vi "Q14070-Z120主界面.vi"() -> ()   [LabVIEW 2013]
uses:
  PCI8622_32.dll
  <vilib>/printing/EasyPrintingControls.llb/report_type.ctl
  <vilib>/Utility/NIReport.llb/NI_ReportGenerationCore.lvlib
  <vilib>/printing/EasyPrintingControls.llb/contents.ctl
  <vilib>/Utility/NIReport.llb/NI_report.lvclass
  <vilib>/printing/EasyPrinting.llb/Easy Print VI Panel or Documentation (path).vi
panel:
  out "电压值":dbl format="%#_4g"
  out "右压力换向(N)":dbl=5000.0 format="%#.2f"
  out "左压力换向(N)":dbl=5000.0 format="%#.2f"
  out "右压力换向":bool
  out "左压力换向":bool
  out "气缸启用":dbl
  in  "型号数量":i32=2
  in  "光幕报警工步":dbl
  out "光幕报警提示":string
  out "顶升压力":dbl
  out "右伺服顶升位置":dbl format="%#.2f"
  out "左伺服顶升位置":dbl format="%#.2f"
  out "右顶升压力合格":bool
  out "左顶升压力合格":bool
  out "保压时间":dbl
  out "error out":errorcluster
  out "右伺服压入深度上限(mm)":dbl format="%#.2f"
  out "右伺服压入深度下限(mm)":dbl format="%#.2f"
  out "右伺服压入力上限(N)":dbl format="%#.2f"
  out "右伺服压入力下限(N)":dbl format="%#.2f"
  out "左伺服压入深度上限(mm)":dbl format="%#.2f"
  out "左伺服压入深度下限(mm)":dbl format="%#.2f"
  out "左伺服压入力上限(N)":dbl format="%#.2f"
  out "左伺服压入力下限(N)":dbl format="%#.2f"
  out "查询上序完成":bool
  out "上序合格":bool
  out "上序完成":bool
  out "本序完成":bool
  out "本序合格":bool
  in  "产品ID字符位数":dbl
  out "压力报警1":bool
  out "压力报警2":bool
  out "伺服慢进速度":dbl
  out "右伺服慢进位置":dbl format="%#.2f"
  out "左伺服慢进位置":dbl format="%#.2f"
  out "JSSJ":string
  out "FGCS":string
  out "KSSJ":string
  out "右压力参数组":dbl[](array[numeric])
  out "右位移参数组":dbl[](array[numeric])
  out "左压力参数组":dbl[](array[numeric])
  out "左位移参数组":dbl[](array[numeric])
  out "右伺服设定走位":dbl
  out "左伺服设定走位":dbl
  out "程序选择-2":bool
  out "程序选择-1":bool
  out "工步提示2":string
  out "工步提示1":string
  in  "报警工步号":u32 caption="工步号1"
  out "报警提示":string
  in  "自动工步号":u32 caption="工步号1"
  out "自动工步提示":string
  in  "产品ID":string="201209190001"
  out "员工ID":string
  out "员工姓名":string
  in  "电动缸全回零":bool
  in  "电动缸全复位":bool
  out "右伺服快进位置":dbl format="%#.2f"
  out "左伺服快进位置":dbl format="%#.2f"
  out "伺服快进速度":dbl
  out "参数保存错误":errorcluster
  out "传感器保存错误":errorcluster
  out "左实时压力(N)":dbl format="%#.3f"
  out "左实时位移(mm)":dbl=10000.0 format="%#.2f"
  out "右实时位移(mm)":dbl=10000.0 format="%#.2f"
  out "右实时压力(N)":dbl format="%#.3f"
  out "区域最小压力(N)":dbl format="%#.3f"
  out "监控点最大压力(N)":dbl format="%#.3f"
  out "监控点最小压力(N)":dbl format="%#.3f"
  out "区域最大压力(N)":dbl format="%#.3f"
  out "区域最小位移(mm)":dbl format="%#.1f"
  out "区域最大位移(mm)":dbl format="%#.1f"
  in  "左工步号2900":u32 caption="工步号1"
  in  "右工步号2700":u32 caption="工步号"
  in  "报警清除":bool
  in  "参数加载":bool
  in  "型号选择":u32(ring) items=["J706", "J709", "J728", "J728A", "J728B", "J506X"]
  out "参数加载错误":errorcluster
  in  "停止":bool
  out "ADODB._Connection Out":refnum<k7>
  out "参数查询错误":errorcluster
  in  "联线按钮":bool
  out "通讯状态":bool
  in  "选项卡控件":T1(tab)
  out "右区域最大压力(N)":dbl
  out "右区域最小压力(N)":dbl
  out "左区域最大压力(N)":dbl
  out "左区域最小压力(N)":dbl
  out "右实测压入压力(N)":dbl format="%#.1f"
  out "左实测压入压力(N)":dbl format="%#.1f"
  out "左压力位移曲线":cluster{"Y":dbl[], "Y":dbl[]}[](graph)=[{"Y"=array[221 elements], "Y"=array[221 elements]}, {"Y"=[130.0, 150.0, 150.0, 130.0, 130.0], "Y"=[0.0, 0.0, 4000.0, 4000.0, 0.0]}] caption="XY图"
  out "右压力位移曲线":cluster{"Y":dbl[], "Y":dbl[]}[](graph)=[{"Y"=array[234 elements], "Y"=array[234 elements]}, {"Y"=[130.0, 150.0, 150.0, 130.0, 130.0], "Y"=[0.0, 0.0, 4000.0, 4000.0, 0.0]}] caption="XY图"
  out "左实测监控点压力(N)":dbl format="%#.3f"
  out "左实测压入位移(mm)":dbl format="%#.1f"
  out "右实测压入位移(mm)":dbl format="%#.1f"
  out "右实测监控点压力(N)":dbl format="%#.3f"
  out "监控点位移(mm)":dbl format="%#.2f"
  out "左压装合格":bool
  out "左压装不合格":bool
  out "右压装不合格":bool
  out "右压装合格":bool
  out "右电动缸零位":bool
  out "左电动缸下限":bool
  out "右气缸下降":bool
  out "右气缸上升":bool
  out "右气缸下位":bool
  out "右气缸上位":bool
  out "左气缸上升":bool
  out "左气缸下降":bool
  out "左气缸上位":bool
  out "左气缸下位":bool
  out "左电动缸零位":bool
  out "右电动缸上限":bool
  out "右电动缸下限":bool
  out "左电动缸上限":bool
  in  "顶升气缸上升-右":bool
  in  "顶升气缸下降-右":bool
  in  "顶升气缸上升-左":bool
  in  "顶升气缸下降-左":bool
  out "启动2按钮":bool
  out "启动1按钮":bool
  out "手动/自动":bool
  out "复位按钮":bool
  in  "电动缸下降-右":bool
  in  "电动缸上升-右":bool
  in  "电动缸下降-左":bool
  in  "电动缸上升-左":bool
  in  "电动缸回零-右":bool
  in  "电动缸回零-左":bool
  in  "电动缸复位-左":bool
  in  "电动缸复位-右":bool
  out "急停按钮":bool
  out "安全光幕":bool
  out "气压报警":bool
  in  "光幕报警使能":bool
  in  "右伺服设定走位":dbl caption="右伺服设定走位负值"
  in  "左伺服设定走位":dbl caption="左伺服设定走位负值"
  in  "电动缸绝对移动调试-右":bool
  in  "电动缸绝对移动调试-左":bool
  out "左伺服实时位置":dbl
  out "右伺服实时位置":dbl
  in  "电动缸复位-右 2":bool
  in  "电动缸复位-左 2":bool
  in  "电动缸回零-左 2":bool
  in  "电动缸回零-右 2":bool
  in  "电动缸下降-右 2":bool
  in  "电动缸上升-右 2":bool
  in  "电动缸下降-左 2":bool
  in  "电动缸上升-左 2":bool
  out "J709减震套批次号输入成功":bool
  out "J706右减震套批次号输入成功":bool
  out "J706左减震套批次号输入成功":bool
  in  "J709减震套批次号":string
  in  "J706右减震套批次号":string
  in  "J706左减震套批次号":string
  in  "传感器参数保存":bool
  in  "压力1零点偏移值":dbl format="%#.3f"
  in  "压力1比例偏移值":dbl format="%#.3f"
  in  "左位移比例偏移值":dbl format="%#.3f"
  in  "左位移零点偏移值":dbl format="%#.3f"
  in  "压力2零点偏移值":dbl format="%#.3f"
  in  "压力2比例偏移值":dbl format="%#.3f"
  in  "右位移比例偏移值":dbl format="%#.3f"
  in  "右位移零点偏移值":dbl format="%#.3f"
  in  "参数保存":bool
  in  "参数查询":bool
  in  "参数列表":string[][](table)
  # "压减震套"
  # "Copying (C) 2014 湖北唯思凌科装备制造有限公司 版权所有"
  # "此界面供伺服定位用，正常生产时 禁止操作！！！"
  # "批次号输入成功"
  # "传感器校验区"
  # "关于传感器校验：\n1、传感器校验需要由具备资质的单位或部门进行校验。\n2、具备权限的用户才能够修改传感器校验参数和试验参数。\n3、修改校验参数方法：先将比例偏移置为1，修改零点偏移，使零点值与校验的传感器一致；然后根据增幅调整比例偏移。"
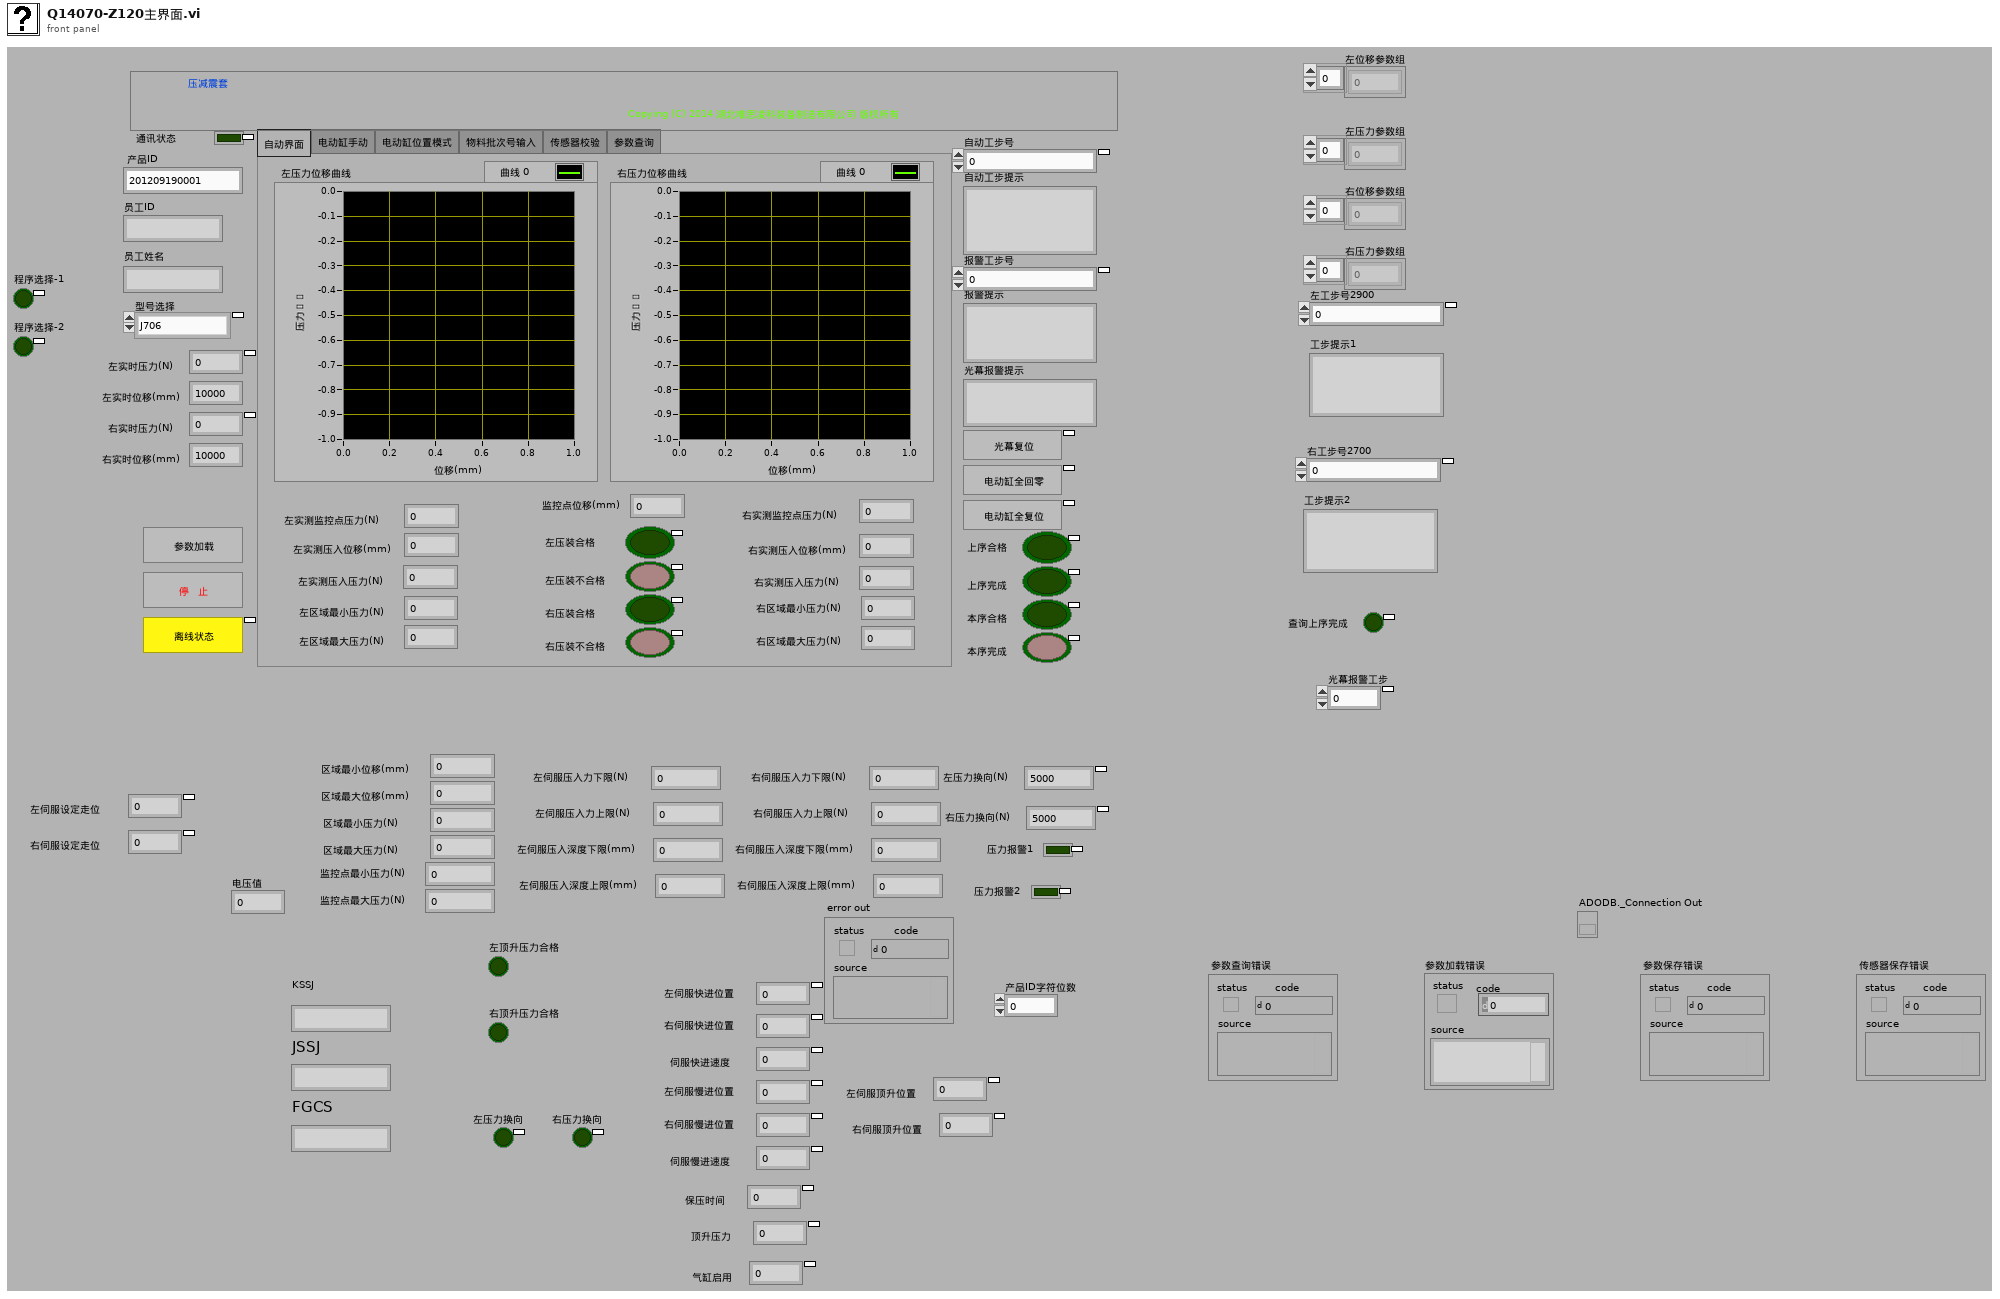
[diagram p1: front panel]
types:
  T1 = enum32{"自动界面", "电动缸手动", "电动缸位置模式", "物料批次号输入", "传感器校验", "参数查询"}
  T2 = enum32{"invalid app kind", "Development System", "Run Time System", "Student Edition", "Embedded LabVIEW", "Evaluation", "Custom"}
  T3 = typedef "NI_ReportGenerationCore.lvlib/report_type.ctl" = u16
  T4 = typedef "NI_ReportGenerationCore.lvlib/contents.ctl" = u16
  T5 = typedef "imagedata.ctl" = cluster{"image type":i32, "image depth":i32, "image":u8[], "mask":u8[], "colors":u32[], "Rectangle":cluster{"left":i16, "top":i16, "right":i16, "bottom":i16}}
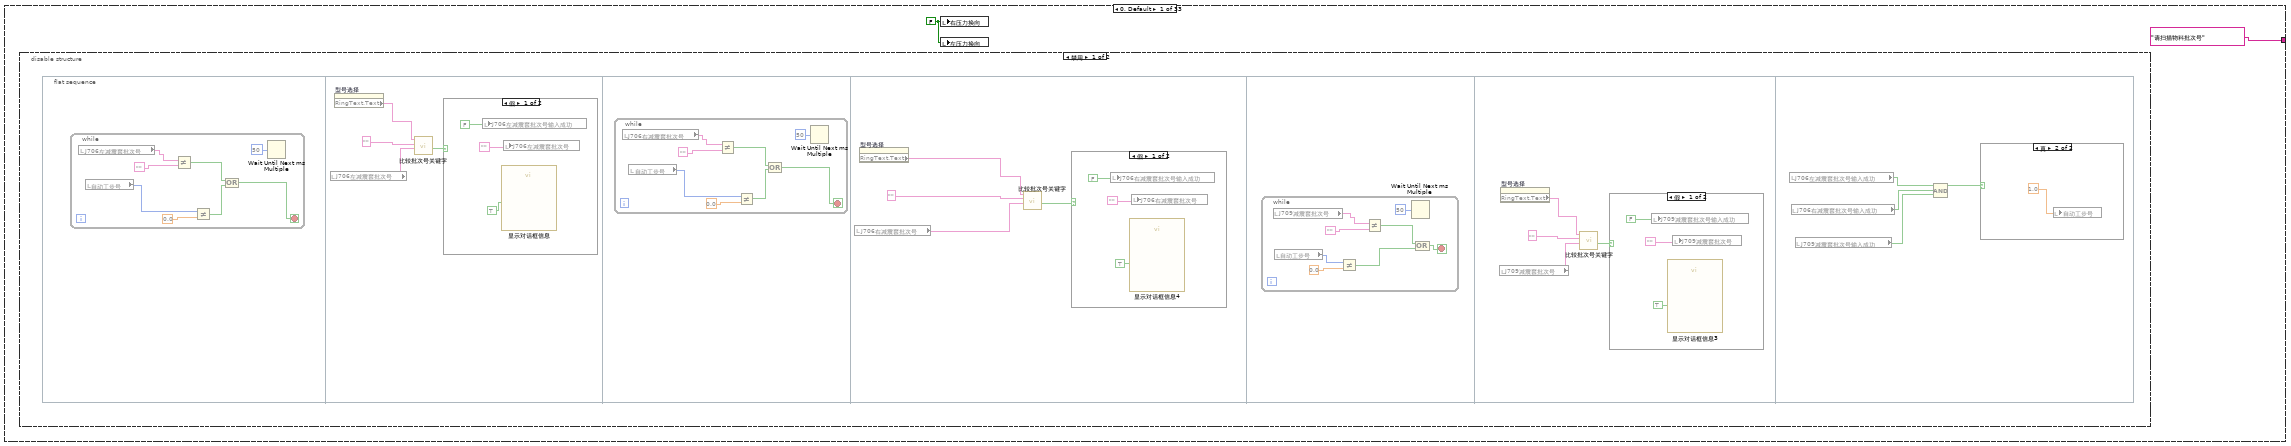
[diagram p3: hidden frame]
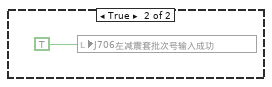
[diagram p4: hidden frame]
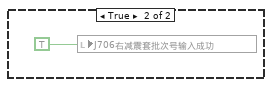
[diagram p5: hidden frame]
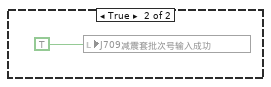
[diagram p6: hidden frame]
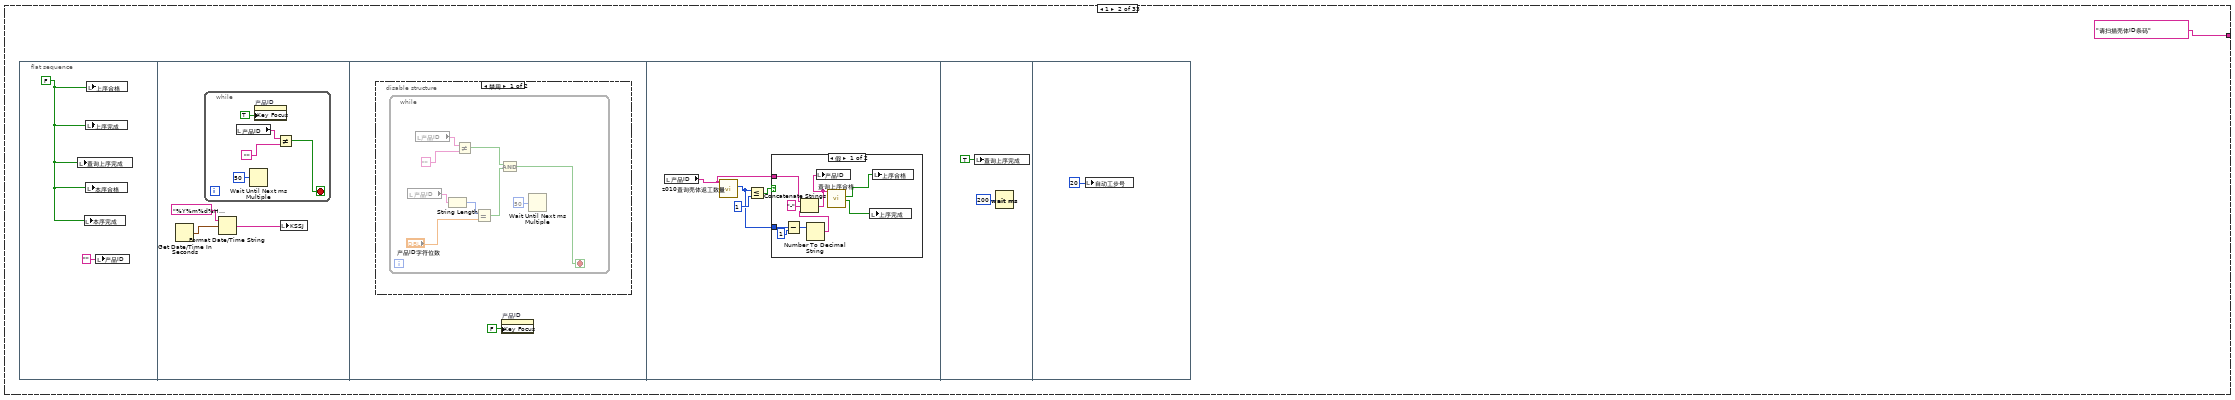
[diagram p9: hidden frame]
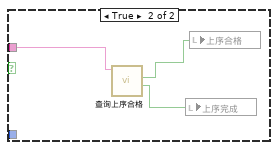
[diagram p11: hidden frame]
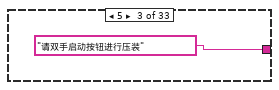
[diagram p12: hidden frame]
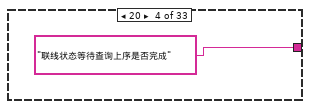
[diagram p13: hidden frame]
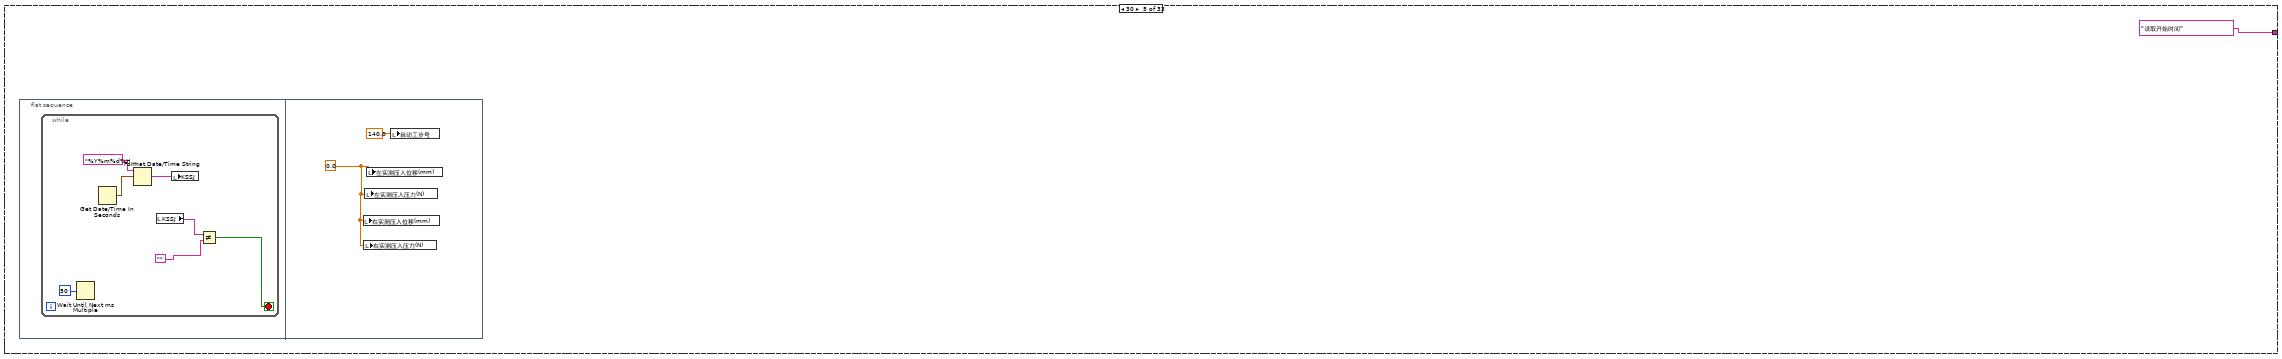
[diagram p14: hidden frame]
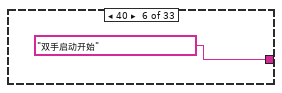
[diagram p15: hidden frame]
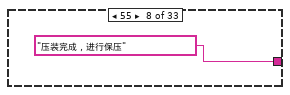
[diagram p16: hidden frame]
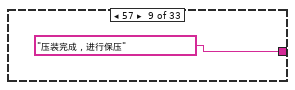
[diagram p17: hidden frame]
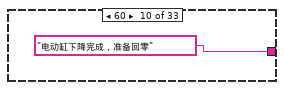
[diagram p18: hidden frame]
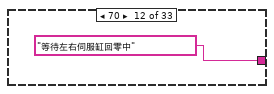
[diagram p20: hidden frame]
diagram:
  n1 = disable-structure shown="禁用" {
    frame Disabled {
      n2 = while {
        stop <- FALSE stop-if-true
        n3 = local read "右实时压力(N)"() -> (w10:dbl)
        n4 = local read "右工步号2700"() -> (w6:u32)
        n5 = local read "左实时压力(N)"() -> (w16:dbl)
        n6 = local read "左工步号2900"() -> (w18:u32)
        n7 = Greater Or Equal?(x=w16, y=1500.0) -> (x >= y?=w13:bool)
        n8 = Equal?(x=w18, y=u32 45) -> (x = y?=w14:bool)
        n9 = Greater Or Equal?(x=w10, y=1500.0) -> (x >= y?=w9:bool)
        n10 = Equal?(x=w6, y=u32 45) -> (x = y?=w5:bool)
        n11 = Compound Arithmetic op=AND(w5, w9) -> (→"右顶升压力合格":bool)
        n12 = Compound Arithmetic op=AND(w14, w13) -> (→"左顶升压力合格":bool)
      }
    }
    frame Enabled {
    }
  }
  n13 = while {
    stop <- w21 stop-if-true
    n14 = Wait Until Next ms Multiple(millisecond multiple=u32 20 ("毫秒倍数")) -> ()  [unwired: 1 out]
    n15 = local read "停止"() -> (w21:bool)
    n16 = local read "左工步号2900"() -> (w19:u32)
    n17 = case shown="20" w19 {
      frame 0, Default {
      }
      frame 20 {
        n18 = flat-sequence {
          tunnel: [w30] -> w22
          tunnel: [w33] -> w24
          tunnel: [w32] -> w23
          tunnel: w22 -> [w31]
          tunnel: w24 -> [w56]
          tunnel: w23 -> [w55]
          frame #0 {
            w25 = FALSE ("压装合格1")
            n19 = local write "左压装不合格"(w25) -> ()
            n20 = local write "左压装合格"(w25) -> ()
          }
          frame #1 {
            n21 = local read "区域最小位移(mm)"() -> (w29:dbl)
            n22 = local read "区域最大位移(mm)"() -> (w28:dbl)
            n23 = local read "区域最小压力(N)"() -> (w27:dbl)
            n24 = local read "区域最大压力(N)"() -> (w26:dbl)
            n25 = call "区域曲线.vi"("区域最大压力(N)"=w26, "区域最小压力(N)"=w27, "区域最大位移(mm)"=w28, "区域最小位移(mm)"=w29) -> ("区域曲线"=w30:cluster{dbl[], dbl[]})  [unwired: 7 in]
          }
          frame #2 {
            w34 = dbl[] []
            n26 = while {
              shift-right: [w51] -> w33
              shift-left: w34 -> [w40]
              shift-right: [w49] -> w32
              shift-left: w34 -> [w50]
              tunnel: w31 -> [w45]
              stop <- w36 stop-if-true
              (unwired) 1 ("索引")
              n27 = shared-variable "我的电脑\\Z120.lvlib\\左实时位置"() -> (w35:dbl)  [unwired: 1 in, 1 out]
              n28 = local read "左压力换向(N)"() -> (w43:dbl)
              n29 = local read "左实时压力(N)"() -> (w42:dbl)
              n30 = shared-variable "我的电脑\\Z120.lvlib\\保护位移"() -> (w39:i16)  [unwired: 1 in, 1 out]
              n31 = local read "左实时位移(mm)"() -> (w48:dbl)
              n32 = local read "左实时压力(N)"() -> (w47:dbl)
              n33 = Negate(x=w35) -> (-x=w41:dbl)
              n34 = Greater Or Equal?(x=w42, y=w43) -> (x >= y?=w37:bool)
              n35 = Build Array (concatenate)(w40, w48) -> (w51:dbl[])
              n36 = Build Array (concatenate)(w50, w47) -> (w49:dbl[])
              n37 = Less Or Equal?(x=w41, y=w39) -> (x <= y?=w38:bool)
              n38 = Or(x=w37, y=w38) -> (x .or. y?=w36:bool)
              n39 = Bundle(w51, w49) -> (w52:cluster{dbl[], dbl[]})  [unwired: 1 in]
              n40 = Build Array(w52, w45) -> (w44:cluster{dbl[], dbl[]}[])
              n41 = local write "左压力位移曲线"(w44) -> ()
              n42 = local write "左压力换向"(w36) -> ()
              n43 = Wait Until Next ms Multiple(millisecond multiple=u32 50 ("毫秒倍数")) -> ()  [unwired: 1 out]
            }
          }
          frame #3 {
            n44 = local read "监控点位移(mm)"() -> (w64:dbl)
            n45 = local read "区域最小压力(N)"() -> (w58:dbl)
            n46 = local read "区域最大压力(N)"() -> (w57:dbl)
            n47 = local read "区域最小位移(mm)"() -> (w60:dbl)
            n48 = local read "区域最大位移(mm)"() -> (w59:dbl)
            n49 = local write "左位移参数组"(w56) -> ()
            n50 = local write "左压力参数组"(w55) -> ()
            n51 = Array Max & Min "数组最大值与最小值"(array=w56) -> (max value=w62:dbl)  [unwired: 3 out]
            n52 = call "压力位移插值.vi"("压力数组"=w55, "监控点位移"=w64, "位移数组"=w56) -> ("监控点压力"=w61:dbl)  [unwired: 2 in]
            n53 = call "区域判断.vi"("压力数组"=w55, "位移数组"=w56, "区域最大压力"=w57, "区域最小压力"=w58, "区域最大位移"=w59, "区域最小位移"=w60) -> ("数值 2"=→"左区域最小压力(N)":dbl, "数值"=→"左区域最大压力(N)":dbl)  [unwired: 1 in, 1 out]
            n54 = local write "左实测监控点压力(N)"(w61) -> ()
            n55 = local write "左实测压入位移(mm)"(w62) -> ()
            n56 = Wait (ms)(milliseconds to wait=u32 200 ("等待时间（毫秒）")) -> ()  [unwired: 1 out]
          }
          frame #4 {
            n57 = local read "左实测压入位移(mm)"() -> (w66:dbl)
            n58 = local read "左位移参数组"() -> (w68:dbl[])
            n59 = local read "左压力参数组"() -> (w67:dbl[])
            n60 = call "压力位移插值.vi"("压力数组"=w67, "监控点位移"=w66, "位移数组"=w68) -> ("监控点压力"=w65:dbl)  [unwired: 2 in]
            n61 = local write "左实测压入压力(N)"(w65) -> ()
          }
          frame #5 {
            n62 = local read "左实测压入压力(N)"() -> (w72:dbl)
            n63 = local read "左伺服压入力下限(N)"() -> (w80:dbl)
            n64 = local read "左伺服压入力上限(N)"() -> (w79:dbl)
            n65 = local read "左伺服压入深度下限(mm)"() -> (w73:dbl)
            n66 = local read "左实测压入位移(mm)"() -> (w69:dbl)
            n67 = local read "左伺服压入深度上限(mm)"() -> (w78:dbl)
            n68 = Less Or Equal?(x=w80, y=w72) -> (x <= y?=w77:bool)
            n69 = Less Or Equal?(x=w72, y=w79) -> (x <= y?=w76:bool)
            n70 = Less Or Equal?(x=w73, y=w69) -> (x <= y?=w75:bool)
            n71 = Less Or Equal?(x=w69, y=w78) -> (x <= y?=w74:bool)
            n72 = Compound Arithmetic op=AND(w77, w76, w75, w74) -> (w71:bool)
            n73 = Not(x=w71) -> (.not. x?=w70:bool)
            n74 = local write "左压装合格"(w71) -> ()
            n75 = local write "左压装不合格"(w70) -> ()
          }
          frame #6 {
            n76 = local write "左工步号2900"(45.0 ("工步2序号")) -> ()
          }
        }
      }
    }
  }
  n77 = while {
    stop <- w84 stop-if-true
    n78 = local read "停止"() -> (w84:bool)
    n79 = Wait Until Next ms Multiple(millisecond multiple=u32 20 ("毫秒倍数")) -> ()  [unwired: 1 out]
    n80 = local read "右工步号2700"() -> (w82:u32)
    n81 = case shown="20" w82 {
      frame 0, Default {
      }
      frame 20 {
        n82 = flat-sequence {
          tunnel: [w89] -> w85
          tunnel: [w96] -> w87
          tunnel: [w95] -> w86
          tunnel: w85 -> [w94]
          tunnel: w87 -> [w119]
          tunnel: w86 -> [w118]
          frame #0 {
            w88 = FALSE ("压装合格2")
            n83 = local write "右压装合格"(w88) -> ()
            n84 = local write "右压装不合格"(w88) -> ()
          }
          frame #1 {
            n85 = local read "区域最小位移(mm)"() -> (w93:dbl)
            n86 = local read "区域最大位移(mm)"() -> (w92:dbl)
            n87 = local read "区域最小压力(N)"() -> (w91:dbl)
            n88 = local read "区域最大压力(N)"() -> (w90:dbl)
            n89 = call "区域曲线.vi"("区域最大压力(N)"=w90, "区域最小压力(N)"=w91, "区域最大位移(mm)"=w92, "区域最小位移(mm)"=w93) -> ("区域曲线"=w89:cluster{dbl[], dbl[]})  [unwired: 7 in]
          }
          frame #2 {
            w97 = dbl[] []
            n90 = while {
              shift-right: [w113] -> w96
              shift-left: w97 -> [w114]
              shift-right: [w111] -> w95
              shift-left: w97 -> [w112]
              tunnel: w94 -> [w108]
              stop <- w98 stop-if-true
              n91 = shared-variable "我的电脑\\Z120.lvlib\\保护位移"() -> (w101:i16)  [unwired: 1 in, 1 out]
              n92 = local read "右实时压力(N)"() -> (w109:dbl)
              n93 = shared-variable "我的电脑\\Z120.lvlib\\右实时位置"() -> (w103:dbl)  [unwired: 1 in, 1 out]
              n94 = local read "右实时位移(mm)"() -> (w106:dbl)
              n95 = local read "右实时压力(N)"() -> (w104:dbl)
              n96 = local read "右压力换向(N)"() -> (w105:dbl)
              n97 = Negate(x=w103) -> (-x=w102:dbl)
              n98 = Build Array (concatenate)(w114, w106) -> (w113:dbl[])
              n99 = Build Array (concatenate)(w112, w109) -> (w111:dbl[])
              n100 = Greater Or Equal?(x=w104, y=w105) -> (x >= y?=w99:bool)
              n101 = Less Or Equal?(x=w102, y=w101) -> (x <= y?=w100:bool)
              n102 = Bundle(w113, w111) -> (w115:cluster{dbl[], dbl[]})  [unwired: 1 in]
              n103 = Or(x=w99, y=w100) -> (x .or. y?=w98:bool)
              n104 = Build Array(w115, w108) -> (w107:cluster{dbl[], dbl[]}[])
              n105 = local write "右压力位移曲线"(w107) -> ()
              n106 = local write "右压力换向"(w98) -> ()
              n107 = Wait Until Next ms Multiple(millisecond multiple=u32 50 ("毫秒倍数")) -> ()  [unwired: 1 out]
            }
          }
          frame #3 {
            n108 = local read "区域最小位移(mm)"() -> (w123:dbl)
            n109 = local read "区域最大位移(mm)"() -> (w122:dbl)
            n110 = local read "监控点位移(mm)"() -> (w126:dbl)
            n111 = local read "区域最小压力(N)"() -> (w121:dbl)
            n112 = local read "区域最大压力(N)"() -> (w120:dbl)
            n113 = local write "右压力参数组"(w118) -> ()
            n114 = local write "右位移参数组"(w119) -> ()
            n115 = Array Max & Min "数组最大值与最小值"(array=w119) -> (max value=w125:dbl)  [unwired: 3 out]
            n116 = call "压力位移插值.vi"("压力数组"=w118, "监控点位移"=w126, "位移数组"=w119) -> ("监控点压力"=w124:dbl)  [unwired: 2 in]
            n117 = call "区域判断.vi"("压力数组"=w118, "位移数组"=w119, "区域最大压力"=w120, "区域最小压力"=w121, "区域最大位移"=w122, "区域最小位移"=w123) -> ("数值 2"=→"右区域最小压力(N)":dbl, "数值"=→"右区域最大压力(N)":dbl)  [unwired: 1 in, 1 out]
            n118 = local write "右实测压入位移(mm)"(w125) -> ()
            n119 = local write "右实测监控点压力(N)"(w124) -> ()
          }
          frame #4 {
            n120 = local read "右实测压入位移(mm)"() -> (w128:dbl)
            n121 = local read "右位移参数组"() -> (w130:dbl[])
            n122 = local read "右压力参数组"() -> (w129:dbl[])
            n123 = call "压力位移插值.vi"("压力数组"=w129, "监控点位移"=w128, "位移数组"=w130) -> ("监控点压力"=w127:dbl)  [unwired: 2 in]
            n124 = local write "右实测压入压力(N)"(w127) -> ()
          }
          frame #5 {
            n125 = local read "右伺服压入力上限(N)"() -> (w136:dbl)
            n126 = local read "右伺服压入深度下限(mm)"() -> (w135:dbl)
            n127 = local read "右伺服压入力下限(N)"() -> (w138:dbl)
            n128 = local read "右实测压入压力(N)"() -> (w137:dbl)
            n129 = local read "右伺服压入深度上限(mm)"() -> (w133:dbl)
            n130 = local read "右实测压入位移(mm)"() -> (w134:dbl)
            n131 = Less Or Equal?(x=w138, y=w137) -> (x <= y?=w139:bool)
            n132 = Less Or Equal?(x=w137, y=w136) -> (x <= y?=w140:bool)
            n133 = Less Or Equal?(x=w135, y=w134) -> (x <= y?=w141:bool)
            n134 = Less Or Equal?(x=w134, y=w133) -> (x <= y?=w142:bool)
            n135 = Compound Arithmetic op=AND(w139, w140, w141, w142) -> (w132:bool)
            n136 = Not(x=w132) -> (.not. x?=w131:bool)
            n137 = local write "右压装不合格"(w131) -> ()
            n138 = local write "右压装合格"(w132) -> ()
          }
          frame #6 {
            n139 = local write "右工步号2700"(45.0 ("工步2序号")) -> ()
          }
        }
      }
    }
  }
  n140 = while {
    stop <- w144 stop-if-true
    n141 = event shown="[1] \"参数查询\": 值改变" {
      selector: _ -> [_ _ _ _ _]
      dyn-events: _ -> [_ _ _ _ _]
      timeout: 200 -> [_ _ _ _ _]
      tunnel: [_ _ _ _ w275] -> w144
      event Timeout {
        n142 = event-data() -> ()  [unwired: 1 in, 3 out]
      }
      event "参数查询": Value Change {
        n143 = event-data() -> ()  [unwired: 1 in, 6 out]
        n144 = flat-sequence {
          tunnel: [w156] -> w147
          tunnel: [w154] -> w146
          tunnel: w147 -> [w160]
          tunnel: w146 -> [w159]
          frame #0 {
            n145 = call "字符串转换为数组.vi"("查询内容"=",产品型号,区域最小位移(mm),区域最大位移(mm),区域最小压力(N),区域最大压力(N),位移监控点(mm),左伺服压入力下限(N),左伺服压入力上限(N),左伺服压入深度下限(mm),左伺服压入深度上限(mm),右伺服压入力下限(N),右伺服压入力上限(N),右伺服压入深度下限(mm),右伺服压入深度上限(mm),左伺服快进位置(mm),右伺服快进位置(mm),伺服快进速度(mm/s),左伺服慢进位置(mm),右伺服慢进位置(mm),左伺服顶升位置(mm),右伺服顶升位置(mm),伺服慢进速度(mm/s),保压时间(ms),顶升压力(N),气缸启用,左压力换向(N),右压力换向(N),伺服模式(0位移，1压力),保护位移,X标尺最小值,X标尺最大值,Y标尺最小值,Y标尺最大值") -> ("列首"=w148:string[])  [unwired: 10 in]
            n146 = property on="参数列表" class="Tbl (严格)"("Row Headers[]"=w148) -> ()  [unwired: 2 in, 2 out]
          }
          frame #1 {
            w153 = 0 ("禁用的索引 (列)")
            n147 = property on="型号选择" class="Ring (严格)"() -> ("RingText.Text"=w150:string)  [unwired: 2 in, 2 out]
            n148 = local read "ADODB._Connection Out"() -> (w157:refnum<k7>)
            n149 = call "创建文本5"("产品型号"=w150) -> ("Result"=w151:string)  [unwired: 13 in, 1 out]
            n150 = call "SQL Execute.vi"("Command Text"=w151, "ADODB._Connection In"=w157) -> ("error out"=w156:errorcluster, "Data"=w158:string[][])  [unwired: 6 in, 2 out]
            n151 = Transpose 2D Array "二维数组转置"(2D array=w158) -> (transposed array=w154:string[][])
            n152 = Index Array(array=w154, index (col)=w153) -> (element=w155:string[])  [unwired: 1 in]
            n153 = Index Array(array=w154, index (col)=w153) -> (element=w152:string[])  [unwired: 1 in]
            n154 = property on="参数列表" class="Tbl (严格)"("Column Headers[]"=w155) -> ()  [unwired: 2 in, 2 out]
            n155 = Array Size(array=w152) -> ()  [unwired: 1 out]
          }
          frame #2 {
            n156 = local write "参数列表"(w159) -> ()
            "参数查询错误" <- w160
          }
        }
      }
      event "参数保存": Value Change {
        n157 = event-data() -> ()  [unwired: 1 in, 6 out]
        n158 = while {
          i -> [w162]
          stop <- w173 stop-if-true
          n159 = local read "型号数量"() -> (w161:i32)
          n160 = local read "参数列表"() -> (w164:string[][])
          n161 = Greater Or Equal?(x=w162, y=w161) -> (x >= y?=w173:bool)
          n162 = Wait Until Next ms Multiple(millisecond multiple=u32 100 ("毫秒倍数")) -> ()  [unwired: 1 out]
          n163 = Index Array "索引数组"(array=w164, index (col)=w162) -> (element=w165:string[])  [unwired: 1 in]
          n164 = stacked-sequence {
            seq-local: [w176 _] -> [_ w238]
            tunnel: w165 -> [w207 w241]
            tunnel: [_ w237] -> w163
            frame #0 {
              n165 = Index Array(array=w207, index #2=1 ("索引"), index #3=2 ("索引"), index #4=3 ("索引"), index #5=4 ("索引"), index #6=5 ("索引"), index #7=6 ("索引"), index #8=7 ("索引"), index #9=8 ("索引"), index #10=9 ("索引"), index #11=10 ("索引"), index #12=11 ("索引"), index #13=12 ("索引"), index #14=13 ("索引"), index #15=14 ("索引"), index #16=15 ("索引"), index #17=16 ("索引"), index #18=17 ("索引"), index #19=18 ("索引"), index #20=19 ("索引"), index #21=20 ("索引"), index #22=21 ("索引"), index #23=22 ("索引"), index #24=23 ("索引")) -> (element #2=w199:string, element #3=w198:string, element #4=w197:string, element #5=w196:string, element #6=w195:string, element #7=w194:string, element #8=w193:string, element #9=w192:string, element #10=w191:string, element #11=w190:string, element #12=w189:string, element #13=w188:string, element #14=w187:string, element #15=w186:string, element #16=w185:string, element #17=w184:string, element #18=w183:string, element #19=w182:string, element #20=w181:string, element #21=w180:string, element #22=w179:string, element #23=w178:string, element #24=w177:string)  [unwired: 2 in, 2 out]
              n166 = call "创建文本3"("区域最小位移"=w199, "区域最a大位移"=w198, "区域最小压力"=w197, "区域最大压力"=w196, "位移监控点"=w195, "左伺服压入力下限"=w194, "左伺服压入力上限"=w193, "左伺服压入深度下限"=w192, "左伺服压入深度上限"=w191, "右伺服压入力下限"=w190, "右伺服压入力上限"=w189, "右伺服压入深度下限"=w188, "右伺服压入深度上限"=w187, "左伺服快进位置"=w186, "右伺服快进位置"=w185, "伺服快进速度"=w184, "左伺服慢进位置"=w183, "右伺服慢进位置"=w182, "左伺服顶升位置"=w181, "右伺服顶升位置"=w180, "伺服慢进速度"=w179, "保压时间"=w178, "顶升压力"=w177) -> ("Result"=w176:string)  [unwired: 3 in, 1 out]
            }
            frame #1 {
              n167 = Index Array(array=w241, index #1=0 ("索引"), index #2=24 ("索引"), index #3=25 ("索引"), index #4=26 ("索引")) -> (element #1=w224:string, element #2=w231:string, element #3=w234:string, element #4=w230:string, element #5=w233:string, element #6=w229:string, element #7=w228:string, element #8=w227:string, element #9=w226:string, element #10=w225:string)  [unwired: 21 in, 15 out]
              n168 = call "创建文本"("气缸启用"=w231, "左压力换向"=w234, "右压力换向"=w230, "伺服模式"=w233, "保护位移"=w229, "X标尺最小值"=w228, "X标尺最大值"=w227, "Y标尺最小值"=w226, "Y标尺最大值"=w225, "产品型号"=w224) -> ("Result"=w232:string)  [unwired: 16 in, 1 out]
              n169 = Concatenate Strings(w238, w232) -> (w237:string)
            }
          }
          n170 = call "ADO Connection Create.vi"() -> ("error out"=w170:errorcluster, "ADODB._Connection Out"=w171:refnum<k7>)  [unwired: 10 in]
          n171 = call "ADO Connection Open.vi"("error in (no error)"=w170, "ConnectionString"="DSN=参数Z120;", "ADODB._Connection In"=w171) -> ("error out"=w167:errorcluster, "ADODB._Connection Out"=w168:refnum<k7>)  [unwired: 7 in]
          n172 = call "SQL Execute.vi"("error in (no error)"=w167, "Command Text"=w163, "ADODB._Connection In"=w168) -> ("error out"=w174:errorcluster, "ADODB._Connection Out"=w175:refnum<k7>)  [unwired: 5 in, 2 out]
          n173 = call "ADO Connection Close.vi"("error in (no error)"=w174, "ADODB._Connection In"=w175) -> ("error out"=→"参数保存错误":errorcluster)  [unwired: 8 in, 1 out]
        }
      }
      event "传感器参数保存": Value Change {
        n174 = event-data() -> ()  [unwired: 1 in, 6 out]
        n175 = local read "左位移零点偏移值"() -> (w267:dbl)
        n176 = local read "左位移比例偏移值"() -> (w268:dbl)
        n177 = local read "右位移零点偏移值"() -> (w271:dbl)
        n178 = local read "右位移比例偏移值"() -> (w272:dbl)
        n179 = local read "压力1零点偏移值"() -> (w265:dbl)
        n180 = local read "压力1比例偏移值"() -> (w266:dbl)
        n181 = local read "压力2零点偏移值"() -> (w269:dbl)
        n182 = local read "压力2比例偏移值"() -> (w270:dbl)
        n183 = Number To Fractional String(number=w265, precision (6)=i16 3 ("精度(6)")) -> (F-format string=w257:string)  [unwired: 2 in]
        n184 = Number To Fractional String(number=w266, precision (6)=i16 3 ("精度(6)")) -> (F-format string=w258:string)  [unwired: 2 in]
        n185 = Number To Fractional String(number=w267, precision (6)=i16 3 ("精度(6)")) -> (F-format string=w259:string)  [unwired: 2 in]
        n186 = Number To Fractional String(number=w268, precision (6)=i16 3 ("精度(6)")) -> (F-format string=w260:string)  [unwired: 2 in]
        n187 = Number To Fractional String(number=w269, precision (6)=i16 3 ("精度(6)")) -> (F-format string=w261:string)  [unwired: 2 in]
        n188 = Number To Fractional String(number=w270, precision (6)=i16 3 ("精度(6)")) -> (F-format string=w262:string)  [unwired: 2 in]
        n189 = Number To Fractional String(number=w271, precision (6)=i16 3 ("精度(6)")) -> (F-format string=w263:string)  [unwired: 2 in]
        n190 = Number To Fractional String(number=w272, precision (6)=i16 3 ("精度(6)")) -> (F-format string=w264:string)  [unwired: 2 in]
        n191 = call "创建文本2"("左位移比例偏移值"=w260, "压力2比例偏移值"=w262, "右位移比例偏移值"=w264, "压力1零点偏移值"=w257, "压力1比例偏移值"=w258, "左位移零点偏移值"=w259, "压力2零点偏移值"=w261, "右位移零点偏移值"=w263) -> ("Result"=w273:string)  [unwired: 6 in, 1 out]
        n192 = call "ADO Connection Create.vi"() -> ("error out"=w246:errorcluster, "ADODB._Connection Out"=w244:refnum<k7>)  [unwired: 10 in]
        n193 = call "ADO Connection Open.vi"("error in (no error)"=w246, "ConnectionString"="DSN=参数Z120;", "ADODB._Connection In"=w244) -> ("error out"=w247:errorcluster, "ADODB._Connection Out"=w245:refnum<k7>)  [unwired: 7 in]
        n194 = call "SQL Execute.vi"("error in (no error)"=w247, "Command Text"=w273, "ADODB._Connection In"=w245) -> ("error out"=w243:errorcluster, "ADODB._Connection Out"=w242:refnum<k7>)  [unwired: 5 in, 2 out]
        n195 = call "ADO Connection Close.vi"("error in (no error)"=w243, "ADODB._Connection In"=w242) -> ("error out"=→"传感器保存错误":errorcluster)  [unwired: 8 in, 1 out]
      }
      event "停止": Value Change {
        n196 = event-data() -> ()  [unwired: 1 in, 6 out]
        n197 = property on="属性节点" class="App"() -> ("App.Kind"=w276:T2)  [unwired: 2 in, 2 out]
        n198 = case shown="\"Development System\"" w276 {
          tunnel: [_ w277 w278] -> w275
          frame "invalid app kind", Default {
          }
          frame "Development System" {
            w277 = TRUE ("停止？(T)")
            n199 = Stop(stop? (T)=w277) -> ()
          }
          frame "Run Time System" {
            w278 = TRUE ("退出？(T)")
            n200 = Quit LabVIEW(quit? (T)=w278) -> ()
          }
        }
      }
    }
  }
  n201 = while {
    stop <- w279 stop-if-true
    n202 = stacked-sequence {
      frame #0 {
        n203 = First Call?() -> (First Call?: T/F=w281:bool)
        n204 = case shown="真" w281 {
          frame False {
          }
          frame True {
            n205 = call "员工管理测试程序.vi"() -> ("员工姓名"=w287:string, "员工ID"=w286:string)  [unwired: 10 in]
            n206 = local write "员工ID"(w286) -> ()
            n207 = local write "员工姓名"(w287) -> ()
          }
        }
        n208 = Negate(x="右伺服设定走位") -> (-x=→"右伺服设定走位":dbl)
        n209 = Negate(x="左伺服设定走位") -> (-x=→"左伺服设定走位":dbl)
      }
      frame #1 {
        n210 = case shown="0, 默认" "报警工步号" {
          tunnel: ["工作正常" "气压报警，请检查气压" "压装过程触碰光幕，请复位后双手启动重新压装" "左压装不合格" "右压装不合格" "左压装压力过大报警" "右压装压力过大报警" "左伺服报警，请复位伺服电机" "右伺服报警，请复位伺服电机" "左伺服达到下极限，请复位后，手动点动上升离开下极限" "左伺服达到上极限，请复位后，手动点动下降离开上极限" "右伺服达到下极限，请复位后，手动点动上升离开下极限" "右伺服达到上极限，请复位后，手动点动下降离开上极限" "联线状态查询上序不合格，请返修"] -> w295
          frame 0, Default {
          }
          frame 1 {
          }
          frame 2 {
          }
          frame 6 {
          }
          frame 7 {
          }
          frame 8 {
          }
          frame 9 {
          }
          frame 11 {
          }
          frame 12 {
          }
          frame 21 {
          }
          frame 22 {
          }
          frame 23 {
          }
          frame 24 {
          }
          frame 41 {
          }
        }
        "报警提示" <- w295
        n211 = case shown="10" "左工步号2900" {
          tunnel: ["准备压装" "左伺服压装启动" "左伺服等待回零完成" "左伺服等待回零完成，等待右伺服回零完成" "左伺服压装中" "左伺服压装结束" "左伺服曲线采集完成" "左伺服回零开始" "左伺服回零中" "左伺服回零完成" "左伺服压装工作结束"] -> w294
          frame 0, Default {
          }
          frame 10 {
          }
          frame 15 {
          }
          frame 16 {
          }
          frame 20 {
          }
          frame 30 {
          }
          frame 40 {
          }
          frame 50 {
          }
          frame 60 {
          }
          frame 70 {
          }
          frame 80 {
          }
        }
        "工步提示1" <- w294
        n212 = case shown="80" "右工步号2700" {
          tunnel: ["准备压装" "右伺服压装启动" "右伺服等待回零完成" "右伺服等待回零完成，等待左伺服回零完成" "右伺服压装中" "右伺服压装结束" "右伺服曲线采集完成" "右伺服回零开始" "右伺服回零中" "右伺服回零完成" "右伺服压装工作结束"] -> w293
          frame 0, Default {
          }
          frame 10 {
          }
          frame 15 {
          }
          frame 16 {
          }
          frame 20 {
          }
          frame 30 {
          }
          frame 40 {
          }
          frame 50 {
          }
          frame 60 {
          }
          frame 70 {
          }
          frame 80 {
          }
        }
        "工步提示2" <- w293
        n213 = case shown="5" "光幕报警工步" {
          tunnel: ["工作正常" "压装过程触碰光幕，请再次启动"] -> w288
          frame 0, Default {
          }
          frame 5 {
          }
        }
        "光幕报警提示" <- w288
        n214 = property on="型号选择" class="Ring (严格)"() -> ("RingText.Text"=w290:string)  [unwired: 2 in, 2 out]
        n215 = case shown="\"J706\", 默认" w290 {
          frame "J706", Default {
            n216 = local write "程序选择-1"(TRUE ("程序选择-1")) -> ()
            n217 = local write "程序选择-2"(FALSE ("程序选择-2")) -> ()
          }
          frame "J709" {
            n218 = local write "程序选择-1"(FALSE ("程序选择-1")) -> ()
            n219 = local write "程序选择-2"(TRUE ("程序选择-2")) -> ()
          }
        }
      }
    }
    n220 = Wait (ms)(milliseconds to wait=u32 50 ("毫秒倍数")) -> ()  [unwired: 1 out]
    n221 = local read "停止"() -> (w279:bool)
  }
  n222 = while {
    stop <- w341 stop-if-true
    n223 = Wait Until Next ms Multiple(millisecond multiple=u32 60 ("毫秒倍数")) -> ()  [unwired: 1 out]
    n224 = local read "自动工步号"() -> (w342:u32)
    n225 = local read "停止"() -> (w341:bool)
    n226 = case shown="50" w342 {
      tunnel: ["请扫描物料批次号" "请扫描壳体ID条码" "请双手启动按钮进行压装" "联线状态等待查询上序是否完成" "读取开始时间" "双手启动开始" "电动缸下降开始" "压装完成，进行保压" "压装完成，进行保压" "电动缸下降完成，准备回零" _ "等待左右伺服缸回零中" "" "" "" "" "" _ "" "" "" "" "" "" "" _ "" "" "" "绘制保存曲线、参数" "上传数据至服务器" "循环完成，归零" "联线状态查询上序不合格，请返修"] -> w339
      frame 0, Default {
        w343 = FALSE ("右压力换向")
        n227 = disable-structure shown="禁用" {
          frame Disabled {
            n228 = flat-sequence {
              frame #0 {
                n229 = while {
                  stop <- w347 stop-if-true
                  n230 = local read "J706左减震套批次号"() -> (w346:string)
                  n231 = local read "自动工步号"() -> (w345:u32)
                  n232 = Not Equal?(x=w346, y="") -> (x != y?=w349:bool)
                  n233 = Not Equal?(x=w345, y=0.0) -> (x != y?=w348:bool)
                  n234 = Compound Arithmetic op=OR(w349, w348) -> (w347:bool)
                  n235 = Wait Until Next ms Multiple(millisecond multiple=u32 50 ("毫秒倍数")) -> ()  [unwired: 1 out]
                }
              }
              frame #1 {
                n236 = local read "J706左减震套批次号"() -> (w355:string)
                n237 = property on="型号选择" class="Ring (严格)"() -> ("RingText.Text"=w353:string)  [unwired: 2 in, 2 out]
                n238 = call "比较批次号关键字.vi"("批次号"=w355, "外购件名称"="", "产品型号"=w353) -> ("关键字正确"=w354:bool)  [unwired: 6 in, 1 out]
                n239 = case shown="假" w354 {
                  frame False {
                    n240 = local write "J706左减震套批次号输入成功"(FALSE ("防尘罩批次号输入成功")) -> ()
                    n241 = call "显示对话框信息"("Enable"=TRUE) -> ()  [unwired: 9 in, 2 out]
                    n242 = local write "J706左减震套批次号"("") -> ()
                  }
                  frame True {
                    n243 = local write "J706左减震套批次号输入成功"(TRUE ("防尘罩批次号输入成功")) -> ()
                  }
                }
              }
              frame #2 {
                n244 = while {
                  stop <- w363 stop-if-true
                  n245 = local read "J706右减震套批次号"() -> (w362:string)
                  n246 = local read "自动工步号"() -> (w361:u32)
                  n247 = Not Equal?(x=w362, y="") -> (x != y?=w365:bool)
                  n248 = Not Equal?(x=w361, y=0.0) -> (x != y?=w364:bool)
                  n249 = Compound Arithmetic op=OR(w365, w364) -> (w363:bool)
                  n250 = Wait Until Next ms Multiple(millisecond multiple=u32 50 ("毫秒倍数")) -> ()  [unwired: 1 out]
                }
              }
              frame #3 {
                n251 = local read "J706右减震套批次号"() -> (w370:string)
                n252 = property on="型号选择" class="Ring (严格)"() -> ("RingText.Text"=w372:string)  [unwired: 2 in, 2 out]
                n253 = call "比较批次号关键字.vi"("批次号"=w370, "外购件名称"="", "产品型号"=w372) -> ("关键字正确"=w371:bool)  [unwired: 6 in, 1 out]
                n254 = case shown="假" w371 {
                  frame False {
                    n255 = local write "J706右减震套批次号输入成功"(FALSE ("防尘罩批次号输入成功")) -> ()
                    n256 = call "显示对话框信息4"("Enable"=TRUE) -> ()  [unwired: 9 in, 2 out]
                    n257 = local write "J706右减震套批次号"("") -> ()
                  }
                  frame True {
                    n258 = local write "J706右减震套批次号输入成功"(TRUE ("防尘罩批次号输入成功")) -> ()
                  }
                }
              }
              frame #4 {
                n259 = while {
                  stop <- w381 stop-if-true
                  n260 = local read "J709减震套批次号"() -> (w380:string)
                  n261 = local read "自动工步号"() -> (w378:u32)
                  n262 = Not Equal?(x=w378, y=0.0) -> (x != y?=w377:bool)
                  n263 = Not Equal?(x=w380, y="") -> (x != y?=w382:bool)
                  n264 = Wait Until Next ms Multiple(millisecond multiple=u32 50 ("毫秒倍数")) -> ()  [unwired: 1 out]
                  n265 = Compound Arithmetic op=OR(w382, w377) -> (w381:bool)
                }
              }
              frame #5 {
                n266 = local read "J709减震套批次号"() -> (w386:string)
                n267 = property on="型号选择" class="Ring (严格)"() -> ("RingText.Text"=w388:string)  [unwired: 2 in, 2 out]
                n268 = call "比较批次号关键字.vi"("批次号"=w386, "外购件名称"="", "产品型号"=w388) -> ("关键字正确"=w387:bool)  [unwired: 6 in, 1 out]
                n269 = case shown="假" w387 {
                  frame False {
                    n270 = local write "J709减震套批次号输入成功"(FALSE ("防尘罩批次号输入成功")) -> ()
                    n271 = call "显示对话框信息3"("Enable"=TRUE) -> ()  [unwired: 9 in, 2 out]
                    n272 = local write "J709减震套批次号"("") -> ()
                  }
                  frame True {
                    n273 = local write "J709减震套批次号输入成功"(TRUE ("防尘罩批次号输入成功")) -> ()
                  }
                }
              }
              frame #6 {
                n274 = local read "J706左减震套批次号输入成功"() -> (w396:bool)
                n275 = local read "J706右减震套批次号输入成功"() -> (w394:bool)
                n276 = local read "J709减震套批次号输入成功"() -> (w393:bool)
                n277 = Compound Arithmetic op=AND(w396, w394, w393) -> (w395:bool)
                n278 = case shown="真" w395 {
                  frame False {
                  }
                  frame True {
                    n279 = local write "自动工步号"(1.0 ("批次号扫描工步")) -> ()
                  }
                }
              }
            }
          }
          frame Enabled {
          }
        }
        n280 = local write "右压力换向"(w343) -> ()
        n281 = local write "左压力换向"(w343) -> ()
      }
      frame 1 {
        n282 = flat-sequence {
          frame #0 {
            w400 = FALSE ("上序合格")
            n283 = local write "查询上序完成"(w400) -> ()
            n284 = local write "本序完成"(w400) -> ()
            n285 = local write "上序完成"(w400) -> ()
            n286 = local write "本序合格"(w400) -> ()
            n287 = local write "上序合格"(w400) -> ()
            n288 = local write "产品ID"("" ("产品ID")) -> ()
          }
          frame #1 {
            n289 = Get Date/Time In Seconds() -> (seconds since 1Jan1904=w403:timestamp)
            n290 = while {
              stop <- w404 stop-if-true
              n291 = local read "产品ID"() -> (w405:string)
              n292 = Wait Until Next ms Multiple(millisecond multiple=u32 50 ("毫秒倍数")) -> ()  [unwired: 1 out]
              n293 = property on="产品ID" class="Str"("Key Focus"=TRUE ("键选中")) -> ()  [unwired: 2 in, 2 out]
              n294 = Not Equal?(x=w405, y="") -> (x != y?=w404:bool)
            }
            n295 = Format Date/Time String(time format string (%c)="%Y%m%d%H%M" ("时间格式字符串(%c)"), seconds (now)=w403) -> (date/time string=w401:string)  [unwired: 1 in]
            n296 = local write "KSSJ"(w401) -> ()
          }
          frame #2 {
            n297 = disable-structure shown="禁用" {
              frame Disabled {
                n298 = while {
                  stop <- w412 stop-if-true
                  n299 = local read "产品ID"() -> (w416:string)
                  n300 = local read "产品ID"() -> (w418:string)
                  n301 = String Length(string=w416) -> (length=w415:i32)
                  n302 = Not Equal?(x=w418, y="") -> (x != y?=w413:bool)
                  n303 = Equal?(x=w415, y="产品ID字符位数") -> (x = y?=w414:bool)
                  n304 = Compound Arithmetic op=AND(w413, w414) -> (w412:bool)
                  n305 = Wait Until Next ms Multiple(millisecond multiple=u32 50 ("毫秒倍数")) -> ()  [unwired: 1 out]
                }
              }
              frame Enabled {
              }
            }
            n306 = property on="产品ID" class="Str"("Key Focus"=FALSE ("键选中")) -> ()  [unwired: 2 in, 2 out]
          }
          frame #3 {
            n307 = local read "产品ID"() -> (w420:string)
            n308 = call "z010查询壳体返工数量.vi"("转向器总成ID"=w420) -> ("Rows Fetched"=w419:i32)  [unwired: 8 in, 2 out]
            n309 = Less Or Equal?(x=w419, y=1) -> (x <= y?=w422:bool)
            n310 = case shown="假" w422 {
              tunnel: w420 -> [w425 w432]
              tunnel: w419 -> [w428 _]
              frame False {
                n311 = Subtract(x=w428, y=1) -> (x-y=w426:i32)
                n312 = Number To Decimal String(number=w426) -> (decimal integer string=w429:string)  [unwired: 1 in]
                n313 = Concatenate Strings(w425, "-" ("字符串"), w429) -> (w423:string)
                n314 = local write "产品ID"(w423) -> ()
                n315 = call "查询上序合格.vi"("产品ID"=w423) -> ("本序已做"=w431:bool, "上序合格"=w430:bool)  [unwired: 8 in, 1 out]
                n316 = local write "上序完成"(w431) -> ()
                n317 = local write "上序合格"(w430) -> ()
              }
              frame True {
                n318 = call "查询上序合格.vi"("产品ID"=w432) -> ("本序已做"=w434:bool, "上序合格"=w433:bool)  [unwired: 8 in, 1 out]
                n319 = local write "上序完成"(w434) -> ()
                n320 = local write "上序合格"(w433) -> ()
              }
            }
          }
          frame #4 {
            n321 = local write "查询上序完成"(TRUE ("查询上序完成")) -> ()
            n322 = Wait (ms)(milliseconds to wait=u32 200 ("等待时间（毫秒）")) -> ()  [unwired: 1 out]
          }
          frame #5 {
            n323 = local write "自动工步号"(u32 20 ("自动工步号")) -> ()
          }
        }
      }
      frame 5 {
      }
      frame 20 {
      }
      frame 30 {
        n324 = flat-sequence {
          frame #0 {
            n325 = while {
              stop <- w441 stop-if-true
              n326 = Wait Until Next ms Multiple(millisecond multiple=u32 50 ("毫秒倍数")) -> ()  [unwired: 1 out]
              n327 = Get Date/Time In Seconds() -> (seconds since 1Jan1904=w446:timestamp)
              n328 = Format Date/Time String(time format string (%c)="%Y%m%d%H%M" ("时间格式字符串(%c)"), seconds (now)=w446) -> (date/time string=w445:string)  [unwired: 1 in]
              n329 = local read "KSSJ"() -> (w443:string)
              n330 = local write "KSSJ"(w445) -> ()
              n331 = Not Equal?(x=w443, y="") -> (x != y?=w441:bool)
            }
          }
          frame #1 {
            w449 = 0.0 ("左实测压入位移(mm)")
            n332 = local write "右实测压入位移(mm)"(w449) -> ()
            n333 = local write "右实测压入压力(N)"(w449) -> ()
            n334 = local write "左实测压入压力(N)"(w449) -> ()
            n335 = local write "左实测压入位移(mm)"(w449) -> ()
            n336 = local write "自动工步号"(140.0 ("内球节工步号")) -> ()
          }
        }
      }
      frame 40 {
      }
      frame 50 {
      }
      frame 55 {
      }
      frame 57 {
      }
      frame 60 {
      }
      frame 65 {
      }
      frame 70 {
      }
      frame 140 {
      }
      frame 150 {
      }
      frame 155 {
      }
      frame 157 {
      }
      frame 160 {
      }
      frame 165 {
      }
      frame 170 {
      }
      frame 180 {
      }
      frame 240 {
      }
      frame 250 {
      }
      frame 255 {
      }
      frame 257 {
      }
      frame 260 {
      }
      frame 265 {
      }
      frame 270 {
      }
      frame 280 {
      }
      frame 290 {
      }
      frame 800 {
        n337 = flat-sequence {
          tunnel: [w501] -> w490
          tunnel: [w499] -> w489
          tunnel: [w493] -> w474
          tunnel: [w491] -> w471
          tunnel: w490 -> [w508]
          tunnel: w489 -> [w507]
          tunnel: [w508] -> w488
          tunnel: [w507] -> w487
          tunnel: ["F:\\报表存储\\" ("字符串")] -> w486
          tunnel: w474 -> [w505]
          tunnel: [w505] -> w473
          tunnel: [w504] -> w472
          tunnel: w471 -> [w504]
          tunnel: w488 -> [w513]
          tunnel: w487 -> [w509]
          tunnel: w486 -> [w514]
          tunnel: [w523] -> w485
          tunnel: [w521] -> w484
          tunnel: [w519] -> w483
          tunnel: [w515] -> w482
          tunnel: w473 -> [w512]
          tunnel: w472 -> [w511]
          tunnel: w485 -> [w529]
          tunnel: [w530] -> w481
          tunnel: w484 -> [w530]
          tunnel: w483 -> [w528]
          tunnel: [w527] -> w480
          tunnel: w482 -> [w526]
          tunnel: [w525] -> w479
          tunnel: [w544] -> w478
          tunnel: w481 -> [w544]
          tunnel: w480 -> [w543]
          tunnel: [w543] -> w477
          tunnel: [w542] -> w476
          tunnel: w479 -> [w542]
          tunnel: w478 -> [w551]
          tunnel: w477 -> [w550]
          tunnel: w476 -> [w547]
          frame #0 {
            n338 = local read "产品ID"() -> (w500:string)
            n339 = Format Date/Time String(time format string (%c)="%Y%m%d" ("时间格式字符串(%c)")) -> (date/time string=w492:string)  [unwired: 2 in]
            n340 = String Subset(string=w492, offset (0)=4 ("偏移量(0)"), length (rest)=2 ("长度（剩余）")) -> (substring=w493:string)
            n341 = String Subset(string=w492, offset (0)=6 ("偏移量(0)"), length (rest)=2 ("长度（剩余）")) -> (substring=w491:string)
            n342 = call <vilib>:"Trim Whitespace.vi"("string"=w500) -> ("trimmed string"=w499:string)  [unwired: 1 in]
            n343 = String Subset(string=w492, offset (0)=0 ("偏移量(0)"), length (rest)=4 ("长度（剩余）")) -> (substring=w501:string)
          }
          frame #1 {
          }
          frame #2 {
            w510 = "\\" ("字符串")
            n344 = Concatenate Strings(w514, w513, w510, w512, w510, w511, w510) -> (w516:string)
            n345 = Concatenate Strings(w514, w513, w510, w512, w510, w511, w510) -> (w524:string)
            n346 = String To Path(string=w524) -> (path=w523:path)
            n347 = Concatenate Strings(w516, w509, ".JPG" ("字符串")) -> (w522:string)
            n348 = Concatenate Strings(w516, w509, "右.txt" ("字符串")) -> (w515:string)
            n349 = Concatenate Strings(w516, w509, "左.txt" ("字符串")) -> (w519:string)
            n350 = String To Path(string=w522) -> (path=w521:path)
          }
          frame #3 {
            n351 = call <vilib>:"Check if File or Folder Exists.vi"("path"=w529) -> ("file or folder exists?"=w531:bool)  [unwired: 8 in, 2 out]
            n352 = String To Path(string=w528) -> (path=w527:path)
            n353 = String To Path(string=w526) -> (path=w525:path)
            n354 = case shown="真" w531 {
              tunnel: w529 -> [w532 w533]
              frame False {
                n355 = Create Folder(path (use dialog)=w532) -> ()  [unwired: 2 in, 3 out]
              }
              frame True {
                n356 = flat-sequence {
                  tunnel: w533 -> [w537]
                  tunnel: [w535] -> w534
                  tunnel: w534 -> [w540]
                  frame #0 {
                    n357 = Delete(path (use dialog)=w537, entire hierarchy (F)=TRUE ("整个层次结构(F)")) -> (deleted path=w535:path)  [unwired: 3 in, 2 out]
                  }
                  frame #1 {
                    n358 = call <vilib>:"Check if File or Folder Exists.vi"("path"=w540) -> ("file or folder exists?"=w539:bool, "dup path"=w538:path)  [unwired: 8 in, 1 out]
                    n359 = case shown="假" w539 {
                      tunnel: w538 -> [w541 _]
                      frame False {
                        n360 = Create Folder(path (use dialog)=w541) -> ()  [unwired: 2 in, 3 out]
                      }
                      frame True {
                      }
                    }
                  }
                }
              }
            }
          }
          frame #4 {
            n361 = Wait Until Next ms Multiple(millisecond multiple=u32 1000 ("毫秒倍数")) -> ()  [unwired: 1 out]
          }
          frame #5 {
            n362 = flat-sequence {
              tunnel: w550 -> [w554]
              tunnel: w551 -> [w555]
              tunnel: [w555] -> w549
              tunnel: [w554] -> w548
              tunnel: w547 -> [w553]
              tunnel: [w553] -> w546
              tunnel: w549 -> [w556]
              tunnel: w548 -> [w559]
              tunnel: w546 -> [w562]
              frame #0 {
                n363 = local write "选项卡控件"(T1."自动界面" ("选项卡控件")) -> ()
              }
              frame #1 {
                n364 = local read "左位移参数组"() -> (w563:dbl[])
                n365 = local read "左压力参数组"() -> (w564:dbl[])
                n366 = local read "右位移参数组"() -> (w560:dbl[])
                n367 = local read "右压力参数组"() -> (w561:dbl[])
                n368 = disable-structure shown="禁用" {
                  disable-tunnel: w556 -> [w565 _]
                  frame Disabled {
                    w568 = T3 2 items=["快速打印", "标准报表", "HTML", "双字节", "Excel"] ("report type (Quick Print)")
                    w567 = T4 1 items=["完整前面板", "前面板可见部分", "图标、说明、前面板和程序框图", "说明信息: 使用前面板", "说明信息: 作为子VI使用", "说明信息: 完整", "说明信息: 自定义"] ("contents (complete front panel)")
                    n369 = Current VI's Path() -> (path=w566:path)
                    n370 = call-poly <vilib>:"Easy Print VI Panel or Documentation.vi"("report type (Quick Print)"=w568, "contents (complete front panel)"=w567, "VI path"=w566) -> ("error out"=w570:errorcluster, "report out"=w569:refnum<class "NI_report.lvclass">)  [unwired: 1 in, 6 out]
                    n371 = call-dynamic "Save Report to File.vi"("report in"=w569, "report file path"=w565, "error in (no error)"=w570) -> ()  [unwired: 2 in, 11 out]
                  }
                  frame Enabled {
                  }
                }
                n372 = call "导出曲线数组.vi"("压力参数"=w564, "位移参数"=w563, "file path (dialog if empty)"=w559) -> ()  [unwired: 17 in]
                n373 = call "导出曲线数组.vi"("压力参数"=w561, "位移参数"=w560, "file path (dialog if empty)"=w562) -> ()  [unwired: 17 in]
                n374 = control-ref of="本VI"() -> (w558:refnum<vi>)
                n375 = invoke class="VI" method="FP.Get Image"(reference=w558) -> ("image data"=w557:T5)  [unwired: 5 in, 5 out]
                n376 = call <vilib>:"Write JPEG File.vi"("image data"=w557, "path to JPEG file"=w556) -> ()  [unwired: 8 in, 2 out]
              }
            }
          }
          frame #6 {
            n377 = local write "自动工步号"(810.0 ("工步号")) -> ()
          }
        }
      }
      frame 810 {
        n378 = flat-sequence {
          tunnel: [w600] -> w573
          tunnel: w573 -> [w608]
          frame #0 {
            n379 = while {
              stop <- w576 stop-if-true
              n380 = Get Date/Time In Seconds() -> (seconds since 1Jan1904=w581:timestamp)
              n381 = local read "JSSJ"() -> (w578:string)
              n382 = Format Date/Time String(time format string (%c)="%Y%m%d%H%M" ("时间格式字符串(%c)"), seconds (now)=w581) -> (date/time string=w579:string)  [unwired: 1 in]
              n383 = Wait Until Next ms Multiple(millisecond multiple=u32 50 ("毫秒倍数")) -> ()  [unwired: 1 out]
              n384 = Not Equal?(x=w578, y="") -> (x != y?=w576:bool)
              n385 = local write "JSSJ"(w579) -> ()
            }
            n386 = Wait (ms)(milliseconds to wait=u32 2000 ("等待时间（毫秒）")) -> ()  [unwired: 1 out]
          }
          frame #1 {
            w598 = i16 4 ("精度(6)")
            n387 = local read "右实测压入位移(mm)"() -> (w588:dbl)
            n388 = local read "右实测压入压力(N)"() -> (w587:dbl)
            n389 = local read "左实测压入压力(N)"() -> (w589:dbl)
            n390 = local read "左实测压入位移(mm)"() -> (w590:dbl)
            n391 = local read "右压装合格"() -> (w582:bool)
            n392 = local read "左压装合格"() -> (w583:bool)
            n393 = local read "J706左减震套批次号"() -> (w593:string)
            n394 = local read "J709减震套批次号"() -> (w591:string)
            n395 = local read "J706右减震套批次号"() -> (w592:string)
            n396 = local read "员工ID"() -> (w604:string)
            n397 = local read "产品ID"() -> (w605:string)
            n398 = local read "KSSJ"() -> (w603:string)
            n399 = local read "JSSJ"() -> (w599:string)
            n400 = local read "FGCS"() -> (w602:string)
            n401 = And(x=w583, y=w582) -> (x .and. y?=w584:bool)
            n402 = Boolean To (0,1)(Boolean=w584) -> (0, 1=w607:i16)
            n403 = Number To Decimal String(number=w607, width (-)=i16 1 ("宽度(-)")) -> (decimal integer string=w585:string)
            n404 = Number To Fractional String(number=w590, precision (6)=w598) -> (F-format string=w597:string)  [unwired: 2 in]
            n405 = Number To Fractional String(number=w589, precision (6)=w598) -> (F-format string=w596:string)  [unwired: 2 in]
            n406 = Number To Fractional String(number=w588, precision (6)=w598) -> (F-format string=w595:string)  [unwired: 2 in]
            n407 = Number To Fractional String(number=w587, precision (6)=w598) -> (F-format string=w594:string)  [unwired: 2 in]
            n408 = Build Array(w605, w604, "1", w585, w603, w599, w602, "Q14070-Z120", w597, w596, w595, w594, w593, w592, w591) -> (w600:string[])
          }
          frame #2 {
            n409 = Wait (ms)(milliseconds to wait=u32 500 ("等待时间（毫秒）")) -> ()  [unwired: 1 out]
            n410 = call "数据库更新.vi"("设备号"="11", "数据"=w608) -> ()  [unwired: 13 in, 1 out]
          }
          frame #3 {
            n411 = local write "自动工步号"(820.0 ("工步号")) -> ()
          }
        }
      }
      frame 820 {
      }
      frame 900 {
      }
    }
    "自动工步提示" <- w339
  }
  n412 = flat-sequence {
    frame #0 {
      n413 = call "ADO Connection Create.vi"() -> ("error out"=w617:errorcluster, "ADODB._Connection Out"=w618:refnum<k7>)  [unwired: 10 in]
      n414 = call "ADO Connection Open.vi"("error in (no error)"=w617, "ConnectionString"="DSN=参数Z120;", "ADODB._Connection In"=w618) -> ("error out"=→"error out":errorcluster, "ADODB._Connection Out"=→"ADODB._Connection Out":refnum<k7>)  [unwired: 7 in]
    }
    frame #1 {
      n415 = while {
        stop <- w620 stop-if-true
        n416 = Wait Until Next ms Multiple(millisecond multiple=u32 100 ("毫秒倍数")) -> ()  [unwired: 1 out]
        n417 = First Call?() -> (First Call?: T/F=w623:bool)
        n418 = Or(x=w623, y="参数加载") -> (x .or. y?=w622:bool)
        n419 = case shown="真" w622 {
          frame False {
          }
          frame True {
            n420 = stacked-sequence {
              frame #0 {
                n421 = First Call?() -> (First Call?: T/F=w624:bool)
                n422 = case shown="真" w624 {
                  frame False {
                  }
                  frame True {
                    n423 = local read "ADODB._Connection Out"() -> (w626:refnum<k7>)
                    n424 = local read "error out"() -> (w625:errorcluster)
                    n425 = call "SQL Execute.vi"("error in (no error)"=w625, "Command Text"="SELECT * FROM 测试参数表 ;", "ADODB._Connection In"=w626) -> ("Data"=w629:string[][])  [unwired: 5 in, 3 out]
                    n426 = Index Array "索引数组"(array=w629, index (col)=0 ("禁用的索引 (列)")) -> (element=w632:string[])  [unwired: 1 in]
                    n427 = Array Size "数组大小"(array=w632) -> (size(s)=w631:i32)
                    n428 = while {
                      shift-right: [w637] -> w630
                      shift-left: i32[] [] -> [w638]
                      tunnel: w631 -> [w635]
                      i -> [w636]
                      stop <- w639 stop-if-true
                      n429 = Greater Or Equal?(x=w636, y=w635) -> (x >= y?=w639:bool)
                      n430 = Build Array (concatenate) "创建数组"(w638, w636) -> (w637:i32[])
                    }
                    n431 = Build Cluster Array "索引与捆绑簇数组"(w632, w630) -> (w627:cluster{"String":string, i32}[])
                    n432 = property on="型号选择" class="Ring (严格)"("StringsAndValues[]"=w627) -> ()  [unwired: 2 in, 2 out]
                  }
                }
              }
              frame #1 {
                n433 = property on="型号选择" class="Ring (严格)"() -> ("RingText.Text"=w644:string)  [unwired: 2 in, 2 out]
                n434 = local read "ADODB._Connection Out"() -> (w642:refnum<k7>)
                n435 = call "创建文本4"("产品型号"=w644) -> ("Result"=w646:string)  [unwired: 13 in, 1 out]
                n436 = local read "error out"() -> (w641:errorcluster)
                n437 = call "SQL Execute.vi"("error in (no error)"=w641, "Command Text"=w646, "ADODB._Connection In"=w642) -> ("error out"=w640:errorcluster, "Data"=w648:string[][])  [unwired: 5 in, 2 out]
                n438 = local write "error out"(w640) -> ()
                n439 = Index Array "索引数组"(array=w648, index (row)=0 ("索引 (行)")) -> (element=w645:string[])  [unwired: 1 in]
                n440 = Fract/Exp String To Number "分数/指数字符串至数值转换"(string=w645) -> (number=w643:dbl[])  [unwired: 3 in, 1 out]
                n441 = stacked-sequence {
                  tunnel: w643 -> [w693 w722]
                  frame #0 {
                    n442 = Index Array(array=w693, index #1=1 ("索引"), index #2=2 ("索引"), index #3=3 ("索引"), index #4=4 ("索引"), index #5=5 ("索引"), index #6=6 ("索引"), index #7=7 ("索引"), index #8=8 ("索引"), index #9=9 ("索引"), index #10=10 ("索引"), index #11=11 ("索引"), index #12=12 ("索引"), index #13=13 ("索引"), index #14=14 ("索引"), index #15=15 ("索引"), index #16=16 ("索引"), index #17=17 ("索引"), index #18=18 ("索引"), index #19=19 ("索引"), index #20=20 ("索引"), index #21=21 ("索引"), index #22=22 ("索引"), index #23=23 ("索引"), index #24=24 ("索引")) -> (element #1=w676:dbl, element #2=w675:dbl, element #3=w674:dbl, element #4=w673:dbl, element #5=w672:dbl, element #6=w671:dbl, element #7=w670:dbl, element #8=w669:dbl, element #9=w668:dbl, element #10=w667:dbl, element #11=w666:dbl, element #12=w665:dbl, element #13=w664:dbl, element #14=w663:dbl, element #15=w662:dbl, element #16=w661:dbl, element #17=w660:dbl, element #18=w659:dbl, element #19=w658:dbl, element #20=w656:dbl, element #21=w654:dbl, element #22=w679:dbl, element #23=→"顶升压力":dbl, element #24=w650:dbl)
                    n443 = To Unsigned Long Integer(number=w679) -> (unsigned 32bit integer=w653:u32)
                    n444 = local write "保压时间"(w653) -> ()
                    n445 = local write "气缸启用"(w650) -> ()
                    n446 = Multiply(x=w663, y=-1.0 ("x")) -> (x*y=w692:dbl)
                    n447 = Multiply(x=w662, y=-1.0) -> (x*y=w691:dbl)
                    n448 = Multiply(x=w660, y=-1.0) -> (x*y=w688:dbl)
                    n449 = Multiply(x=w659, y=-1.0 ("x")) -> (x*y=w686:dbl)
                    n450 = Multiply(x=w658, y=-1.0 ("x")) -> (x*y=w657:dbl)
                    n451 = Multiply(x=w656, y=-1.0 ("x")) -> (x*y=w655:dbl)
                    n452 = local write "区域最小位移(mm)"(w676) -> ()
                    n453 = local write "区域最大位移(mm)"(w675) -> ()
                    n454 = local write "区域最小压力(N)"(w674) -> ()
                    n455 = local write "区域最大压力(N)"(w673) -> ()
                    n456 = local write "监控点位移(mm)"(w672) -> ()
                    n457 = local write "左伺服压入力下限(N)"(w671) -> ()
                    n458 = local write "左伺服压入力上限(N)"(w670) -> ()
                    n459 = local write "左伺服压入深度下限(mm)"(w669) -> ()
                    n460 = local write "左伺服压入深度上限(mm)"(w668) -> ()
                    n461 = local write "右伺服压入力下限(N)"(w667) -> ()
                    n462 = local write "右伺服压入力上限(N)"(w666) -> ()
                    n463 = local write "右伺服压入深度下限(mm)"(w665) -> ()
                    n464 = local write "右伺服压入深度上限(mm)"(w664) -> ()
                    n465 = local write "左伺服快进位置"(w692) -> ()
                    n466 = local write "右伺服快进位置"(w691) -> ()
                    n467 = local write "伺服快进速度"(w661) -> ()
                    n468 = local write "左伺服慢进位置"(w688) -> ()
                    n469 = local write "右伺服慢进位置"(w686) -> ()
                    n470 = local write "左伺服顶升位置"(w657) -> ()
                    n471 = local write "右伺服顶升位置"(w655) -> ()
                    n472 = local write "伺服慢进速度"(w654) -> ()
                  }
                  frame #1 {
                    n473 = Index Array(array=w722, index #1=25 ("索引"), index #2=26 ("索引")) -> (element #1=→"左压力换向(N)":dbl, element #2=→"右压力换向(N)":dbl, element #3=w717:dbl, element #4=w716:dbl, element #5=w714:dbl, element #6=w713:dbl, element #7=w712:dbl, element #8=w711:dbl)  [unwired: 13 in, 7 out]
                    n474 = property on="右压力位移曲线" class="XYGraph (严格)"("XScale.Maximum"=w713) -> ()  [unwired: 2 in, 2 out]
                    n475 = property on="左压力位移曲线" class="XYGraph (严格)"("XScale.Maximum"=w713) -> ()  [unwired: 2 in, 2 out]
                    n476 = property on="右压力位移曲线" class="XYGraph (严格)"("XScale.Minimum"=w714) -> ()  [unwired: 2 in, 2 out]
                    n477 = property on="左压力位移曲线" class="XYGraph (严格)"("XScale.Minimum"=w714) -> ()  [unwired: 2 in, 2 out]
                    n478 = property on="右压力位移曲线" class="XYGraph (严格)"("YScale.Maximum"=w711) -> ()  [unwired: 2 in, 2 out]
                    n479 = property on="左压力位移曲线" class="XYGraph (严格)"("YScale.Minimum"=w712) -> ()  [unwired: 2 in, 2 out]
                    n480 = property on="右压力位移曲线" class="XYGraph (严格)"("YScale.Minimum"=w712) -> ()  [unwired: 2 in, 2 out]
                    n481 = property on="左压力位移曲线" class="XYGraph (严格)"("YScale.Maximum"=w711) -> ()  [unwired: 2 in, 2 out]
                    n482 = Negate(x=w716) -> (-x=w715:dbl)
                    n483 = shared-variable "我的电脑\\Z120.lvlib\\保护位移"(w715) -> ()  [unwired: 1 in, 1 out]
                    n484 = shared-variable "我的电脑\\Z120.lvlib\\伺服模式"(w717) -> ()  [unwired: 1 in, 1 out]
                  }
                }
              }
              frame #2 {
                n485 = local read "ADODB._Connection Out"() -> (w735:refnum<k7>)
                n486 = call "SQL Execute.vi"("Command Text"="SELECT * FROM 传感器校验表 where ID='2'", "ADODB._Connection In"=w735) -> ("Data"=w736:string[][])  [unwired: 6 in, 3 out]
                n487 = Index Array "索引数组"(array=w736) -> (element=w737:string[])  [unwired: 2 in]
                n488 = Fract/Exp String To Number "分数/指数字符串至数值转换"(string=w737) -> (number=w738:dbl[])  [unwired: 3 in, 1 out]
                n489 = Index Array "索引数组"(array=w738, index #1=1 ("索引"), index #2=2 ("索引"), index #3=3 ("索引"), index #4=4 ("索引"), index #5=5 ("索引"), index #6=6 ("索引"), index #7=7 ("索引"), index #8=8 ("索引")) -> (element #1=w730:dbl, element #2=w729:dbl, element #3=w728:dbl, element #4=w727:dbl, element #5=w726:dbl, element #6=w725:dbl, element #7=w724:dbl, element #8=w723:dbl)
                n490 = local write "左位移零点偏移值"(w728) -> ()
                n491 = local write "左位移比例偏移值"(w727) -> ()
                n492 = local write "右位移零点偏移值"(w724) -> ()
                n493 = local write "右位移比例偏移值"(w723) -> ()
                n494 = local write "压力1零点偏移值"(w730) -> ()
                n495 = local write "压力1比例偏移值"(w729) -> ()
                n496 = local write "压力2零点偏移值"(w726) -> ()
                n497 = local write "压力2比例偏移值"(w725) -> ()
              }
            }
          }
        }
        n498 = local read "停止"() -> (w620:bool)
      }
    }
    frame #2 {
      n499 = local read "ADODB._Connection Out"() -> (w744:refnum<k7>)
      n500 = call "ADO Connection Close.vi"("ADODB._Connection In"=w744) -> ("error out"=→"参数加载错误":errorcluster)  [unwired: 9 in, 1 out]
    }
  }
  n501 = flat-sequence {
    tunnel: [w746] -> w3
    tunnel: w3 -> [w748]
    tunnel: [w747] -> w2
    tunnel: w2 -> [w822]
    tunnel: [w822] -> w1
    tunnel: w1 -> [w824]
    frame #0 {
      n502 = call "PCI8622配置.vi"() -> ("DeviceID"=w746:i32)  [unwired: 11 in]
    }
    frame #1 {
      n503 = while {
        tunnel: w748 -> [w784]
        tunnel: [w784] -> w747
        stop <- w775 stop-if-true
        w820 = 0  # nRetSizeWords
        w821 = 2048  # nReadSizeWords
        # "hDevice"
        n504 = Wait Until Next ms Multiple(millisecond multiple=u32 2 ("毫秒倍数")) -> ()  [unwired: 1 out]
        n505 = Initialize Array(u16 0, 2048 ("dimension size")) -> (w813:u16[])
        n506 = dll-call lib="PTH17abs FQ14070-Z120人机界面-Z120PCI8622_32.dll" fn="PCI8622_ReadDeviceProAD_Npt" label="ReadDeviceProAD_Npt"("hDevice"=w784, "ADBuffer[]"=w813, "nReadSizeWords"=w821, "nRetSizeWords"=w820) -> ("ADBuffer[]"=w816:u16[])  [unwired: 7 in, 2 out]
        n507 = Divide(x=w816, y=65536.01) -> (x/y=w817:dbl[])
        n508 = Multiply(x=w817, y=20) -> (x*y=w761:dbl[])
        n509 = Subtract(x=w761, y=10) -> (x-y=w762:dbl[])
        n510 = Decimate 1D Array "抽取一维数组"(w762) -> (w810:dbl[], w799:dbl[], w789:dbl[], w788:dbl[])
        n511 = Add Array Elements(numeric array=w789) -> (sum=w786:dbl)
        n512 = Add Array Elements(numeric array=w810) -> (sum=w759:dbl)
        n513 = Array Size(array=w789) -> (size(s)=w798:i32)
        n514 = Add Array Elements(numeric array=w799) -> (sum=w805:dbl)
        n515 = Array Size(array=w810) -> (size(s)=w811:i32)
        n516 = Array Size(array=w799) -> (size(s)=w806:i32)
        n517 = Add Array Elements(numeric array=w788) -> (sum=w785:dbl)
        n518 = Array Size(array=w788) -> (size(s)=w787:i32)
        n519 = Divide(x=w786, y=w798) -> (x/y=w797:dbl)
        n520 = Divide(x=w759, y=w811) -> (x/y=w758:dbl)
        "电压值" <- w758
        n521 = Divide(x=w805, y=w806) -> (x/y=w803:dbl)
        n522 = Divide(x=w785, y=w787) -> (x/y=w793:dbl)
        n523 = local read "压力1零点偏移值"() -> (w769:dbl)
        n524 = Subtract(x=w797, y=-0.02) -> (x-y=w779:dbl)
        n525 = local read "右位移零点偏移值"() -> (w766:dbl)
        n526 = Subtract(x=w803, y=0.49) -> (x-y=w801:dbl)
        n527 = Subtract(x=w793, y=0.0) -> (x-y=w777:dbl)
        n528 = Subtract(x=w758, y=-0.156) -> (x-y=w808:dbl)
        n529 = local read "压力2零点偏移值"() -> (w772:dbl)
        n530 = local read "左位移零点偏移值"() -> (w768:dbl)
        n531 = Multiply(x=w801, y=1000.0) -> (x*y=w800:dbl)
        n532 = Multiply(x=w808, y=1000.0) -> (x*y=w807:dbl)
        n533 = Subtract(x=w800, y=w769) -> (x-y=w763:dbl)
        n534 = Multiply(x=w777, y=25.0) -> (x*y=w790:dbl)
        n535 = Multiply(x=w779, y=25.0) -> (x*y=w794:dbl)
        n536 = local read "压力1比例偏移值"() -> (w770:dbl)
        n537 = Subtract(x=w807, y=w772) -> (x-y=w764:dbl)
        n538 = local read "右位移比例偏移值"() -> (w765:dbl)
        n539 = Subtract(x=w790, y=w768) -> (x-y=w776:dbl)
        n540 = Subtract(x=w794, y=w766) -> (x-y=w778:dbl)
        n541 = local read "压力2比例偏移值"() -> (w771:dbl)
        n542 = local read "左位移比例偏移值"() -> (w767:dbl)
        n543 = Multiply(x=w763, y=w770) -> (x*y=w755:dbl)
        n544 = Multiply(x=w778, y=w765) -> (x*y=w774:dbl)
        n545 = local write "右实时位移(mm)"(w774) -> ()
        n546 = shared-variable "我的电脑\\Z120.lvlib\\左实时压力"() -> (w752:sgl[])  [unwired: 1 in, 1 out]
        n547 = Multiply(x=w764, y=w771) -> (x*y=w756:dbl)
        n548 = Multiply(x=w776, y=w767) -> (x*y=w773:dbl)
        n549 = Greater Or Equal?(x=w755, y=20000.0) -> (x >= y?=→"压力报警2":bool)
        n550 = local write "左实时压力(N)"(w756) -> ()
        n551 = shared-variable "我的电脑\\Z120.lvlib\\右实时压力"() -> (w750:sgl[])  [unwired: 1 in, 1 out]
        n552 = local write "右实时压力(N)"(w755) -> ()
        n553 = Replace Array Subset(array=w752, new element=w756, index=0 ("索引")) -> (w753:sgl[])
        n554 = local write "左实时位移(mm)"(w773) -> ()
        n555 = Greater Or Equal?(x=w756, y=20000.0) -> (x >= y?=→"压力报警1":bool)
        n556 = shared-variable "我的电脑\\Z120.lvlib\\左实时压力"(w753) -> ()  [unwired: 1 in, 1 out]
        n557 = Replace Array Subset(array=w750, new element=w755, index=0 ("索引")) -> (w749:sgl[])
        n558 = shared-variable "我的电脑\\Z120.lvlib\\右实时压力"(w749) -> ()  [unwired: 1 in, 1 out]
        n559 = local read "停止"() -> (w775:bool)
      }
    }
    frame #2 {
      n560 = dll-call lib="PTH17abs FQ14070-Z120人机界面-Z120PCI8622_32.dll" fn="PCI8622_StopDeviceProAD" label="StopDeviceProAD"("hDevice"=w822) -> ("hDevice"=w823:i32)  [unwired: 4 in, 2 out]
      n561 = dll-call lib="PTH17abs FQ14070-Z120人机界面-Z120PCI8622_32.dll" fn="PCI8622_ReleaseDeviceProAD" label="ReleaseDeviceProAD"("hDevice"=w823) -> ()  [unwired: 5 in, 2 out]
    }
    frame #3 {
      n562 = dll-call lib="PTH17abs FQ14070-Z120人机界面-Z120PCI8622_32.dll" fn="PCI8622_ReleaseDevice" label="ReleaseDevice"("hDevice"=w824) -> ()  [unwired: 5 in, 2 out]
    }
  }
